vi "Check Valid.vi"(11 "IReference.lvclass":refnum<class "IReference.lvclass">) -> (3 "Valid?":bool)   [LabVIEW 2019, in "IReference.lvclass"]
uses:
  IReference.lvclass
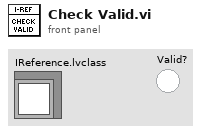
[diagram p1: front panel]
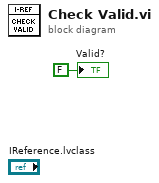
[diagram p0: block diagram]
diagram:
  "Valid?" <- FALSE ("Valid?")
